vi "Update GPU Graph.vi"(6 "f0":dbl, 8 "error in (no error)":errorcluster, 9 "df":dbl, 10 "Plot":sgl[](array[numeric]), 11 "Simple UI in":refnum<class "Simple UI.lvclass">) -> (0 "error out":errorcluster, 3 "Simple UI out":refnum<class "Simple UI.lvclass">)   [LabVIEW 2020, in "Simple UI.lvlib" / "Simple UI.lvclass"]
uses:
  Simple UI.lvclass
  Simple UI.lvclass/Simple UI.ctl
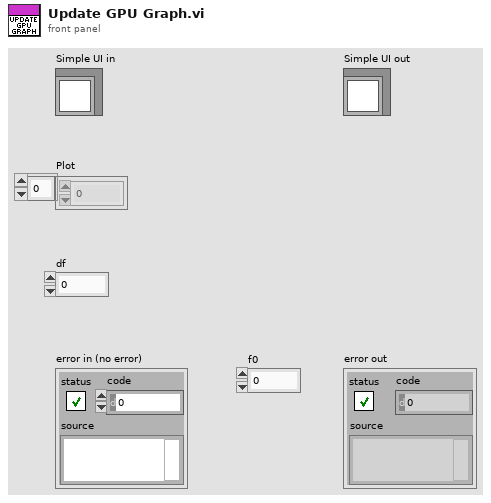
[diagram p1: front panel]
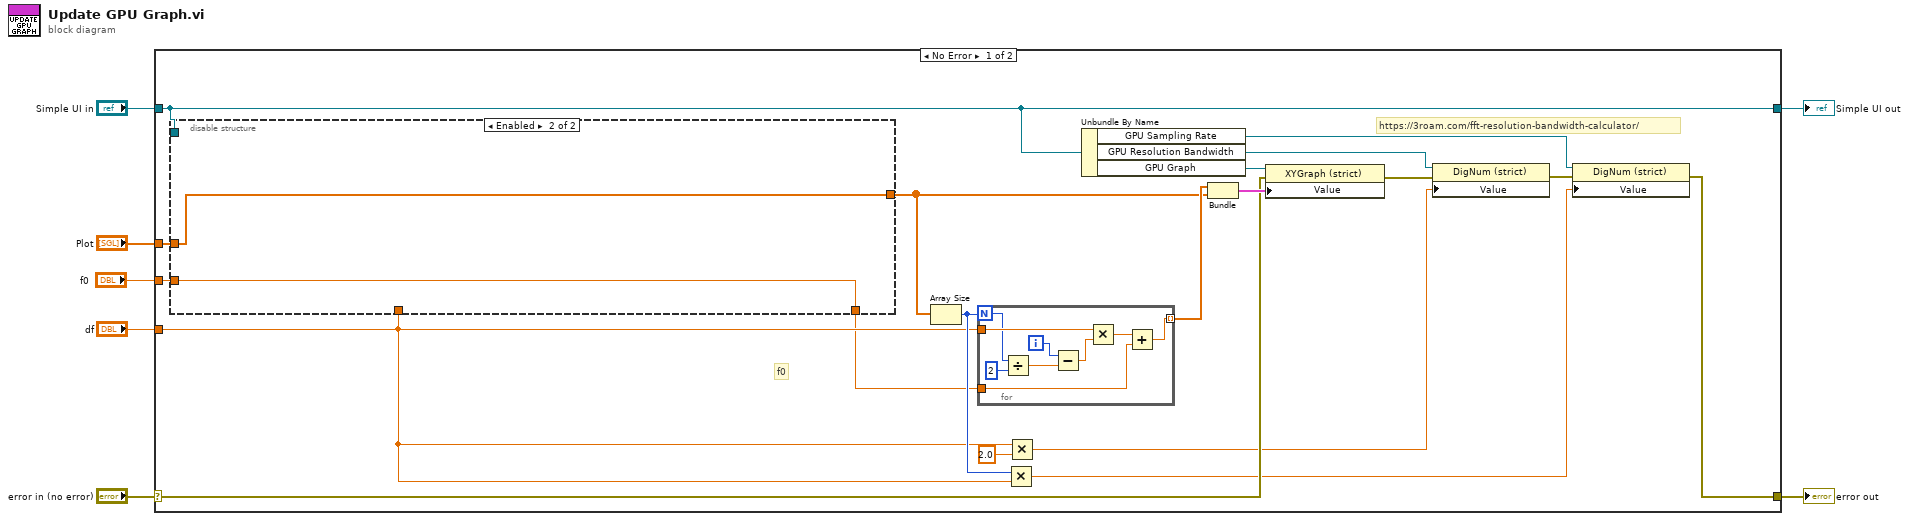
[diagram p0: block diagram]
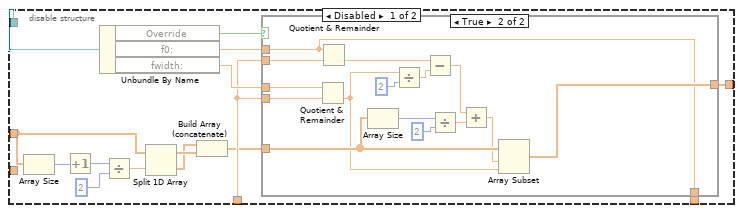
[diagram p2: hidden frame]
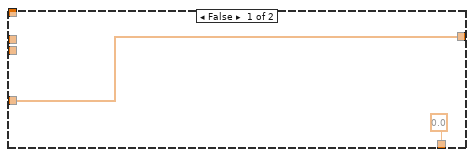
[diagram p3: hidden frame]
diagram:
  n1 = case shown="No Error" "error in (no error)" {
    selector: "error in (no error)" -> [w24 w71]
    tunnel: [w18 w71] -> w3
    tunnel: [w15 w70] -> w2
    tunnel: "Simple UI in" -> [w15 w70]
    tunnel: "Plot" -> [w9 _]
    tunnel: "df" -> [w14 _]
    tunnel: "f0" -> [w8 _]
    frame No Error {
      # "f0"
      # "https://3roam.com/fft-resolution-bandwidth-calculator/"
      n2 = disable-structure shown="Enabled" {
        disable-tunnel: w15 -> [w41 _]
        disable-tunnel: w14 -> [w37 _]
        disable-tunnel: [w36 w60] -> w13
        disable-tunnel: [w35 w59] -> w12
        disable-tunnel: w9 -> [w34 w60]
        disable-tunnel: w8 -> [_ w59]
        frame Disabled {
          n3 = Array Size(array=w34) -> (size(s)=w33:i32)
          n4 = Increment(x=w33) -> (x+1=w31:i32)
          n5 = Unbundle By Name(w41) -> ("Override"=w39:bool, "f0:"=w40:dbl, "fwidth:"=w38:dbl)
          n6 = Divide(x=w31, y=2) -> (x/y=w32:dbl)
          n7 = Split 1D Array(array=w34, index=w32) -> (first subarray=w29:sgl[], second subarray=w28:sgl[])
          n8 = Build Array (concatenate)(w28, w29) -> (w27:sgl[])
          n9 = case shown="True" w39 {
            tunnel: w40 -> [_ w44]
            tunnel: w38 -> [_ w58]
            tunnel: w37 -> [_ w57]
            tunnel: w37 -> [_ w56]
            tunnel: [w43 w55] -> w36
            tunnel: w27 -> [w43 w54]
            tunnel: [0.0 w44] -> w35
            frame False {
            }
            frame True {
              n10 = Quotient & Remainder(x=w58, y=w57) -> (floor(x/y)=w47:dbl)  [unwired: 1 out]
              n11 = Quotient & Remainder(x=w44, y=w56) -> (floor(x/y)=w52:dbl)  [unwired: 1 out]
              n12 = Array Size(array=w54) -> (size(s)=w53:i32)
              n13 = Divide(x=w47, y=2) -> (x/y=w45:dbl)
              n14 = Subtract(x=w52, y=w45) -> (x-y=w46:dbl)
              n15 = Divide(x=w53, y=2) -> (x/y=w49:dbl)
              n16 = Add(x=w46, y=w49) -> (x+y=w50:dbl)
              n17 = Array Subset(array=w54, index=w50, length=w47) -> (w55:sgl[])
            }
          }
        }
        frame Enabled {
        }
      }
      n18 = Array Size(array=w13) -> (size(s)=w16:i32)
      n19 = for {
        N: w16 -> [w68]
        tunnel: w14 -> [w69]
        tunnel: [w61] -> w26 mode=indexing
        tunnel: w12 -> [w64]
        i -> [w66]
        n20 = Divide(x=w68, y=2) -> (x/y=w65:dbl)
        n21 = Subtract(x=w66, y=w65) -> (x-y=w63:dbl)
        n22 = Multiply(x=w69, y=w63) -> (x*y=w62:dbl)
        n23 = Add(x=w62, y=w64) -> (x+y=w61:dbl)
      }
      n24 = Multiply(x=w16, y=w14) -> (x*y=w17:dbl)
      n25 = Multiply(x=w14, y=2.0) -> (x*y=w11:dbl)
      n26 = Unbundle By Name(w15) -> ("GPU Sampling Rate"=w19:refnum<vi>, "GPU Resolution Bandwidth"=w21:refnum<vi>, "GPU Graph"=w23:refnum<vi>)
      n27 = Bundle(w26, "Plot"=w13) -> (w25:cluster{dbl[], "Plot":sgl[]})  [unwired: 1 in]
      n28 = property class="XYGraph (strict)"(reference=w23, error in=w24, "Value"=w25) -> (error out=w22:errorcluster)  [unwired: 1 out]
      n29 = property class="DigNum (strict)"(reference=w21, error in=w22, "Value"=w11) -> (error out=w20:errorcluster)  [unwired: 1 out]
      n30 = property class="DigNum (strict)"(reference=w19, error in=w20, "Value"=w17) -> (error out=w18:errorcluster)  [unwired: 1 out]
    }
    frame Error {
    }
  }
  "error out" <- w3
  "Simple UI out" <- w2
